vi "TCPIP_AcquisitionChA.vi"() -> ()   [LabVIEW 2018]
panel:
  out "error out 5":errorcluster
  out "error out":errorcluster
  in  "stop":bool
  out "error out 4":errorcluster
  in  "Cluster":T1
  out "error out 3":errorcluster
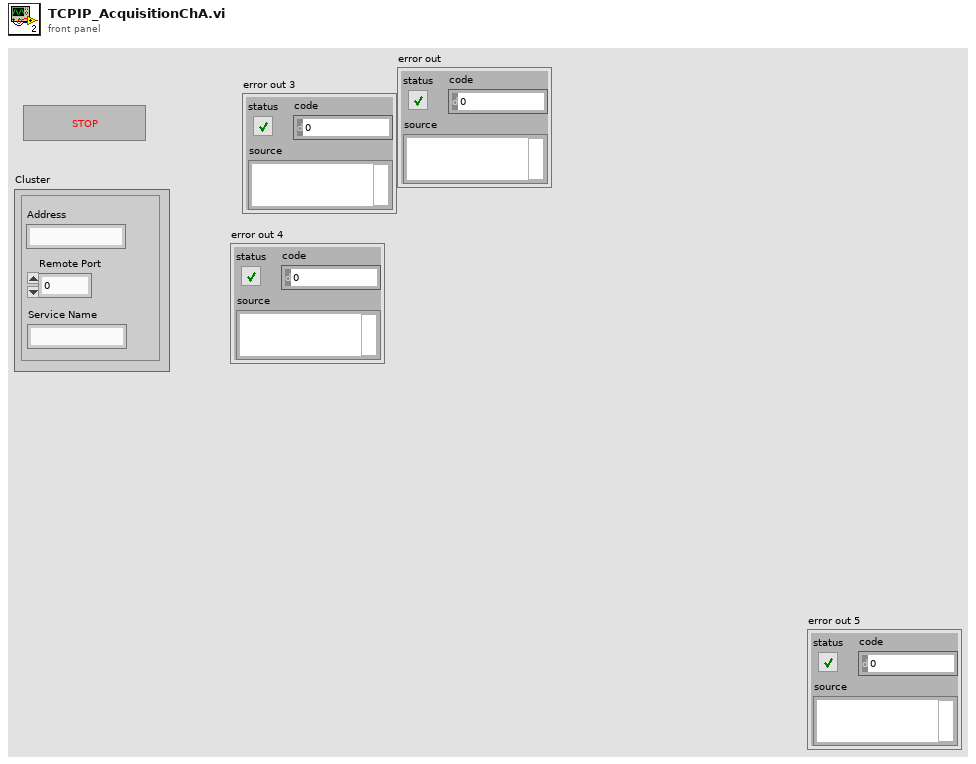
[diagram p1: front panel]
types:
  T1 = cluster{"Address":string, "Remote Port":u32, "Service Name":string}
  T2 = enum16{"Standard", "Buffered", "CRLF", "Immediate"}
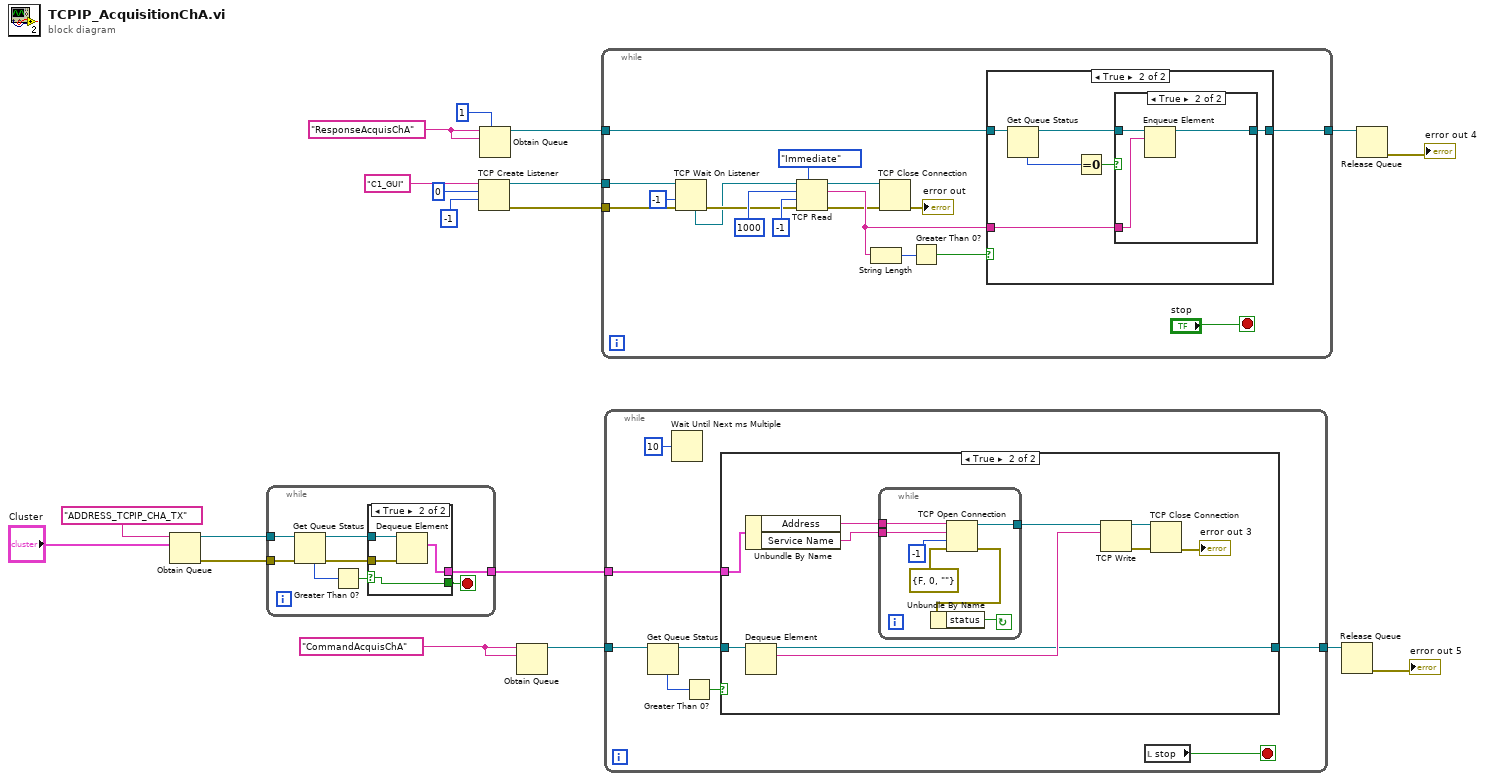
[diagram p0: block diagram]
diagram:
  w10 = "ResponseAcquisChA"
  w13 = "CommandAcquisChA"
  n1 = Obtain Queue(name (unnamed)="ADDRESS_TCPIP_CHA_TX", element data type="Cluster") -> (queue out=w15:refnum<queue>, error out=w16:errorcluster)  [unwired: 3 in, 1 out]
  n2 = while {
    tunnel: [w27] -> w17
    tunnel: w16 -> [w25]
    tunnel: w15 -> [w24]
    stop <- w20 stop-if-true
    n3 = Get Queue Status(queue=w24, error in (no error)=w25) -> (queue out=w23:refnum<queue>, error out=w26:errorcluster, # elements in queue=w22:i32)  [unwired: 1 in, 5 out]
    n4 = Greater Than 0?(x=w22) -> (x > 0?=w21:bool)
    n5 = case shown="True" w21 {
      selector: w21 -> [w28 w29]
      tunnel: [_ w32] -> w27
      tunnel: w26 -> [_ w31]
      tunnel: w23 -> [_ w30]
      tunnel: [w28 w29] -> w20
      frame False {
      }
      frame True {
        n6 = Dequeue Element(queue=w30, error in (no error)=w31) -> (element=w32:T1)  [unwired: 1 in, 3 out]
      }
    }
  }
  n7 = TCP Create Listener(9:-1 ("timeout ms (25000)"), 10:u16 0 ("port"), 11:"C1_GUI" ("service name")) -> (0:w5:errorcluster, 3:w6:refnum<k5>)  [unwired: 2 in, 1 out]
  n8 = Obtain Queue(max queue size (-1, unlimited)=1, name (unnamed)=w10, element data type=w10) -> (queue out=w12:refnum<queue>)  [unwired: 2 in, 2 out]
  n9 = Obtain Queue(name (unnamed)=w13, element data type=w13) -> (queue out=w19:refnum<queue>)  [unwired: 3 in, 2 out]
  n10 = while {
    tunnel: w12 -> [w48]
    tunnel: w6 -> [w41]
    tunnel: w5 -> [w38]
    tunnel: [w35] -> w4
    stop <- "stop" stop-if-true
    n11 = TCP Wait On Listener(8:w38, 9:-1 ("timeout ms (wait forever: -1)"), 11:w41) -> (0:w37:errorcluster, 4:w33:refnum<k5>)  [unwired: 1 in, 3 out]
    n12 = TCP Read(connection ID=w33, bytes to read=1000, error in (no error)=w37, 7:T2."Immediate" ("mode (standard)"), 9:-1 ("bytes to read")) -> (connection ID out=w40:refnum<k5>, data out=w45:string, error out=w39:errorcluster)
    n13 = String Length(string=w45) -> (length=w47:i32)
    n14 = TCP Close Connection(connection ID=w40, error in (no error)=w39) -> (error out=→"error out":errorcluster)  [unwired: 1 in, 1 out]
    n15 = Greater Than 0?(x=w47) -> (x > 0?=w46:bool)
    n16 = case shown="True" w46 {
      tunnel: w48 -> [w50 w54]
      tunnel: w45 -> [_ w52]
      tunnel: [w50 w51] -> w35
      frame False {
      }
      frame True {
        n17 = Get Queue Status(queue=w54) -> (queue out=w53:refnum<queue>, # elements in queue=w56:i32)  [unwired: 2 in, 6 out]
        n18 = Equal To 0?(x=w56) -> (x = 0?=w55:bool)
        n19 = case shown="True" w55 {
          tunnel: w53 -> [w57 w60]
          tunnel: w52 -> [_ w59]
          tunnel: [w57 w58] -> w51
          frame False {
          }
          frame True {
            n20 = Enqueue Element(queue=w60, element=w59) -> (queue out=w58:refnum<queue>)  [unwired: 2 in, 2 out]
          }
        }
      }
    }
  }
  n21 = while {
    tunnel: w19 -> [w68]
    tunnel: w17 -> [w64]
    tunnel: [w61] -> w1
    stop <- w62 stop-if-true
    n22 = Get Queue Status(queue=w68) -> (queue out=w65:refnum<queue>, # elements in queue=w67:i32)  [unwired: 2 in, 6 out]
    n23 = Wait Until Next ms Multiple(millisecond multiple=u32 10 ("milliseconds to wait")) -> ()  [unwired: 1 out]
    n24 = Greater Than 0?(x=w67) -> (x > 0?=w66:bool)
    n25 = case shown="True" w66 {
      tunnel: w65 -> [w69 w79]
      tunnel: w64 -> [_ w77]
      tunnel: [w69 w73] -> w61
      frame False {
      }
      frame True {
        n26 = Unbundle By Name(w77) -> ("Address"=w75:string, "Service Name"=w74:string)
        n27 = Dequeue Element(queue=w79) -> (queue out=w73:refnum<queue>, element=w78:string)  [unwired: 2 in, 2 out]
        n28 = while {
          tunnel: [w86] -> w76
          tunnel: w75 -> [w85]
          tunnel: w74 -> [w80]
          stop <- w81 continue-if-true
          n29 = TCP Open Connection(address=w85, remote port or service name=w80, timeout ms (60000)=-1, error in (no error)=errorcluster {"status"=FALSE, "code"=0, "source"=""}) -> (connection ID=w86:refnum<k5>, error out=w82:errorcluster)  [unwired: 1 in]
          n30 = Unbundle By Name(w82) -> ("status"=w81:bool)
        }
        n31 = TCP Write(connection ID=w76, data in=w78) -> (connection ID out=w70:refnum<k5>, error out=w72:errorcluster)  [unwired: 2 in, 1 out]
        n32 = TCP Close Connection(connection ID=w70, error in (no error)=w72) -> (error out=→"error out 3":errorcluster)  [unwired: 1 in, 1 out]
      }
    }
    n33 = local read "stop"() -> (w62:bool)
  }
  n34 = Release Queue(queue=w1) -> (error out=→"error out 5":errorcluster)  [unwired: 2 in, 2 out]
  n35 = Release Queue(queue=w4) -> (error out=→"error out 4":errorcluster)  [unwired: 2 in, 2 out]
